vi "Get_RegData_String.vi"(8 "error in (no error)":errorcluster, 11 "Class in":refnum<class "IB_RegData_String.lvclass">) -> (0 "error out":errorcluster, 2 "string":string, 3 "Class out":refnum<class "IB_RegData_String.lvclass">)   [LabVIEW 2020, in "IB_RegData_String.lvclass"]
uses:
  <vilib>/AppBuilder/IB_Classes/RegData/RegData_String/IB_RegData_String.lvclass
  <vilib>/AppBuilder/IB_Classes/RegData/RegData_String/IB_RegData_String.lvclass/IB_RegData_String.ctl
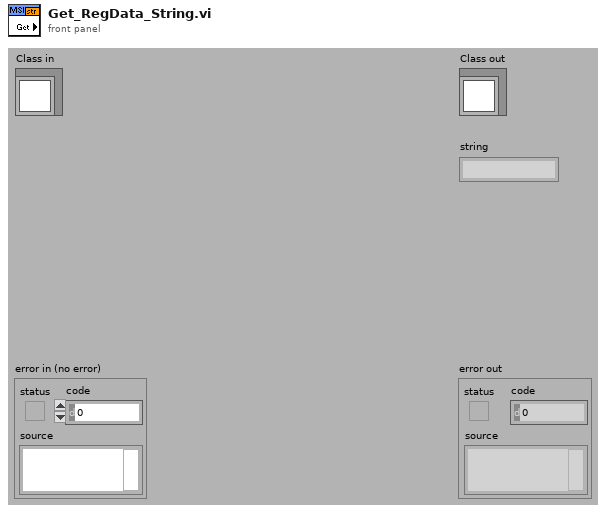
[diagram p1: front panel]
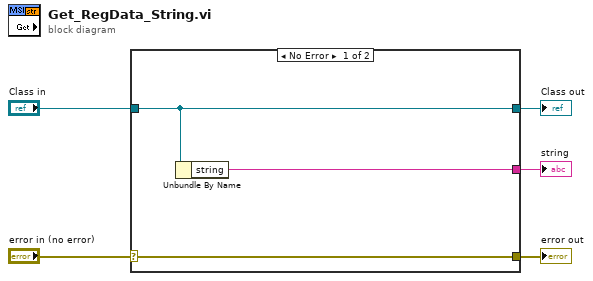
[diagram p0: block diagram]
diagram:
  n1 = case shown="No Error" "error in (no error)" {
    selector: "error in (no error)" -> [w8 w9]
    tunnel: [w8 w9] -> w4
    tunnel: [w7 w10] -> w2
    tunnel: "Class in" -> [w7 w10]
    tunnel: [w6 _] -> w1
    frame No Error {
      n2 = Unbundle By Name(w7) -> ("string"=w6:string)
    }
    frame Error {
    }
  }
  "error out" <- w4
  "Class out" <- w2
  "string" <- w1
